vi "XIPIN_3GPP_LTE_MIMO_Decoder_2_1.vi"   [LabVIEW 2017]
doc: "The 3GPP LTE MIMO Decoder LogiCORE is a drop-in module for Virtex-5(TM), Virtex-6(TM), Virtex-6L(TM), Virtex-7(TM) and Kintex-7(TM) families of FPGA. It performs MIMO decoding using the MMSE algorithm. The core is fully synchronous, using a single clock, and integrates seamlessly with the Xilinx design flow.\n------------------------------------\n<b>Need License</b> : Yes"
uses:
  <vilib>/rvi/XilinxIP/XIPIN_XNode/niFpgaXIPIN.xnode
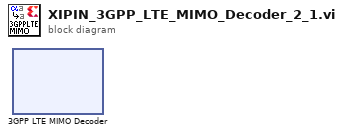
[diagram p0: block diagram]
diagram:
  n1 = xnode ("3GPP LTE MIMO Decoder")() -> ()
